vi "setDevice.vi"(8 "error in (no error)":errorcluster, 9 "device.lvclass":refnum<class "device.lvclass">, 10 "index":i32, 11 "DeviceArray.lvclass in":refnum<class "DeviceArray.lvclass">) -> (0 "error out":errorcluster, 3 "DeviceArray.lvclass out":refnum<class "DeviceArray.lvclass">)   [LabVIEW 2009, in "Tools.lvlib" / "DatabaseHelpers.lvlib" / "DeviceArray.lvclass"]
uses:
  DeviceArray.lvclass
  device/device.lvclass
  DeviceArray.lvclass/DeviceArray.ctl
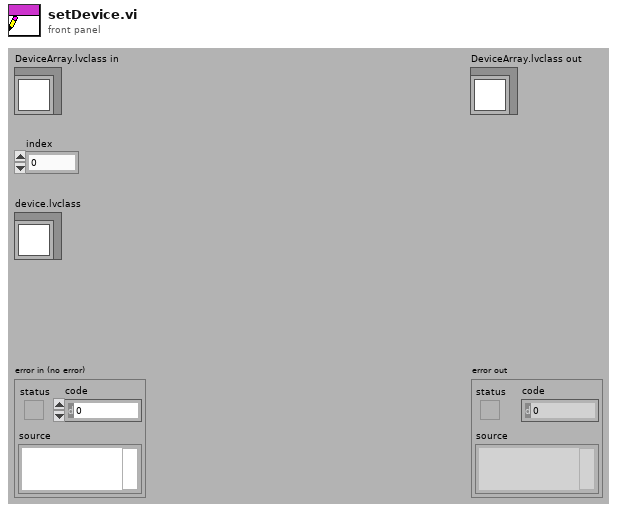
[diagram p1: front panel]
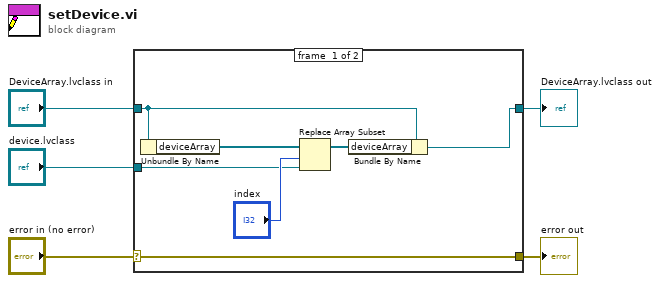
[diagram p0: block diagram]
diagram:
  n1 = case shown="No Error" "error in (no error)" {
    selector: "error in (no error)" -> [w12 w13]
    tunnel: [w12 w13] -> w4
    tunnel: [w11 w14] -> w2
    tunnel: "DeviceArray.lvclass in" -> [w10 w14]
    tunnel: "device.lvclass" -> [w6 _]
    frame #0 {
      n2 = Unbundle By Name(w10) -> ("deviceArray"=w9:refnum<class "device.lvclass">[])
      n3 = Replace Array Subset(array=w9, new element=w6, index="index") -> (w8:refnum<class "device.lvclass">[])
      n4 = Bundle By Name(cluster=w10, "deviceArray"=w8) -> (w11:refnum<class "DeviceArray.lvclass">)
    }
    frame #1 {
    }
  }
  "error out" <- w4
  "DeviceArray.lvclass out" <- w2
